vi "ASCII_To_Hex.vi"(11 "ASCII String":string) -> (0 "hex 4":u8, 1 "hex 3":u8, 2 "hex 2":u8, 3 "hex1":u8, 5 "hex数组":u16[](array[numeric]) format="%x")   [LabVIEW 2018]
panel:
  out "hex5":u8
  out "hex6":u8
  out "hex 7":u8
  out "hex 8":u8
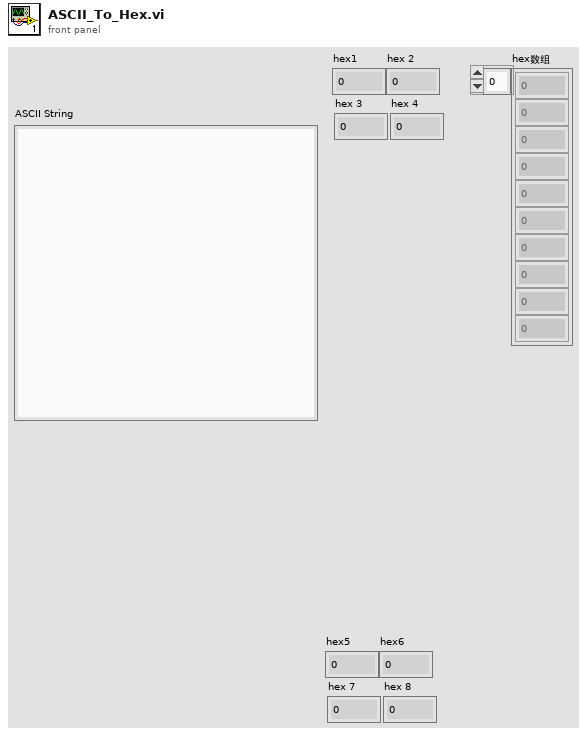
[diagram p1: front panel]
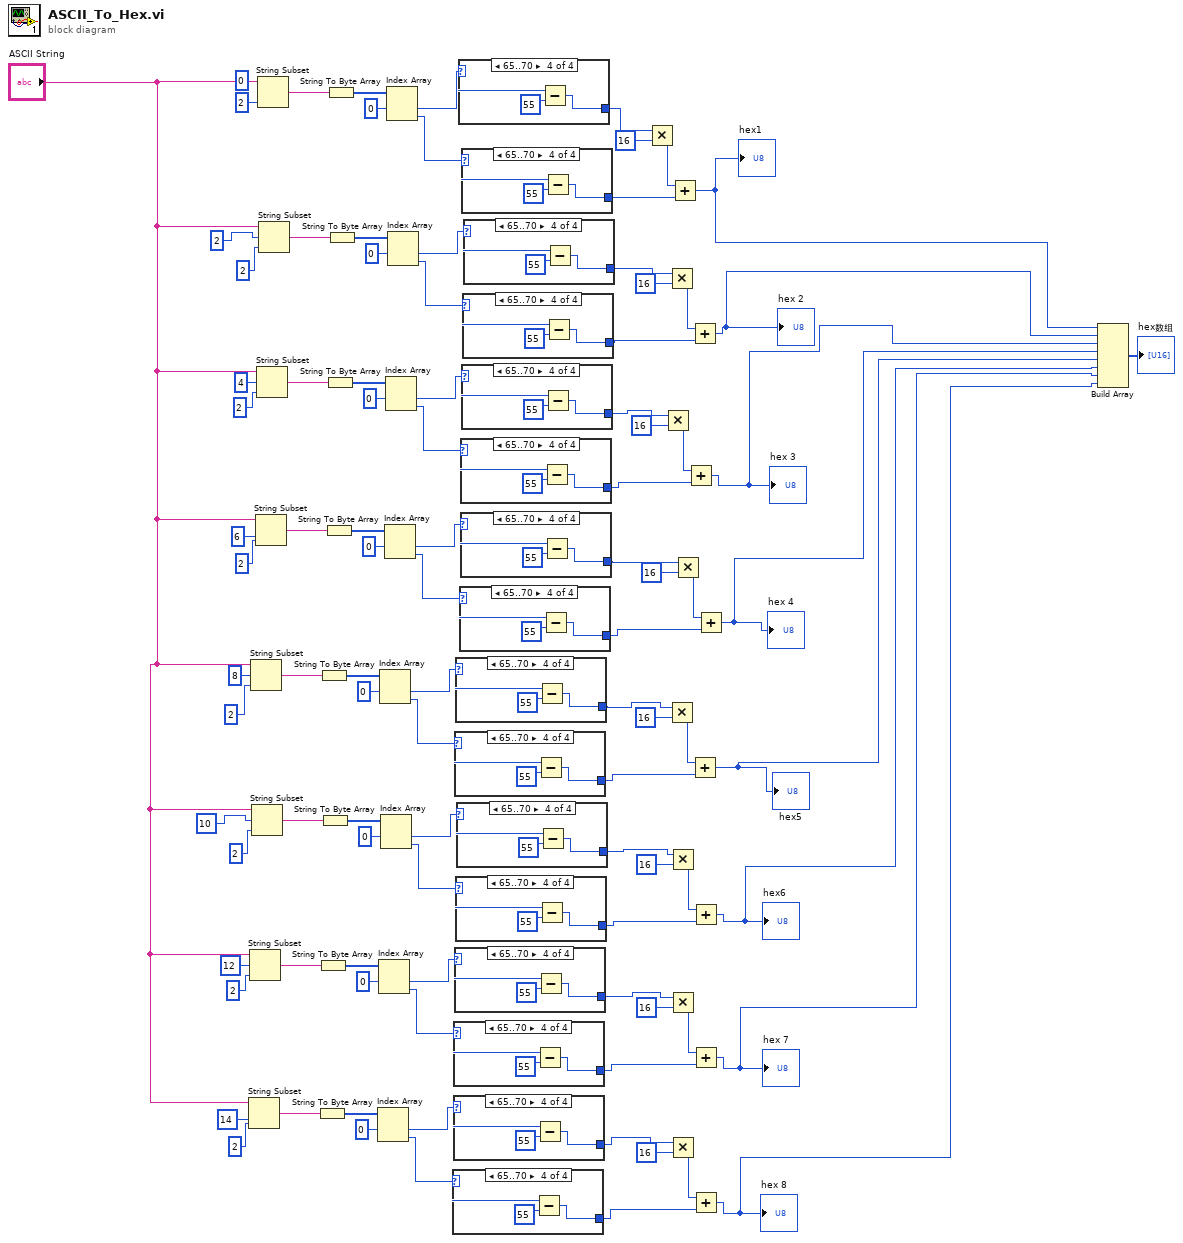
[diagram p0: block diagram]
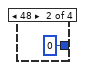
[diagram p3: hidden frame]
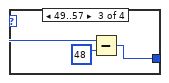
[diagram p4: hidden frame]
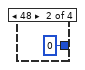
[diagram p6: hidden frame]
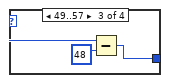
[diagram p7: hidden frame]
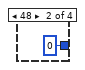
[diagram p9: hidden frame]
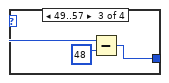
[diagram p10: hidden frame]
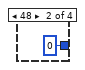
[diagram p12: hidden frame]
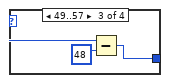
[diagram p13: hidden frame]
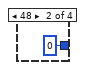
[diagram p15: hidden frame]
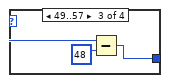
[diagram p16: hidden frame]
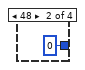
[diagram p18: hidden frame]
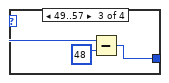
[diagram p19: hidden frame]
diagram:
  n1 = String Subset(string="ASCII String", offset (0)=14 ("偏移量(0)"), length (rest)=2 ("长度（剩余）")) -> (substring=w67:string)
  n2 = String Subset(string="ASCII String", offset (0)=12 ("偏移量(0)"), length (rest)=2 ("长度（剩余）")) -> (substring=w58:string)
  n3 = String Subset(string="ASCII String", offset (0)=8 ("偏移量(0)"), length (rest)=2 ("长度（剩余）")) -> (substring=w46:string)
  n4 = String Subset(string="ASCII String", offset (0)=10 ("偏移量(0)"), length (rest)=2 ("长度（剩余）")) -> (substring=w55:string)
  n5 = String Subset(string="ASCII String", offset (0)=6 ("偏移量(0)"), length (rest)=2 ("长度（剩余）")) -> (substring=w76:string)
  n6 = String Subset(string="ASCII String", offset (0)=4 ("偏移量(0)"), length (rest)=2 ("长度（剩余）")) -> (substring=w85:string)
  n7 = String Subset(string="ASCII String", offset (0)=0 ("偏移量(0)"), length (rest)=2 ("长度（剩余）")) -> (substring=w97:string)
  n8 = String Subset(string="ASCII String", offset (0)=2 ("偏移量(0)"), length (rest)=2 ("长度（剩余）")) -> (substring=w88:string)
  n9 = String To Byte Array(string=w67) -> (unsigned byte array=w66:u8[])
  n10 = String To Byte Array(string=w58) -> (unsigned byte array=w59:u8[])
  n11 = String To Byte Array(string=w46) -> (unsigned byte array=w47:u8[])
  n12 = String To Byte Array(string=w55) -> (unsigned byte array=w54:u8[])
  n13 = String To Byte Array(string=w76) -> (unsigned byte array=w77:u8[])
  n14 = String To Byte Array(string=w85) -> (unsigned byte array=w84:u8[])
  n15 = String To Byte Array(string=w97) -> (unsigned byte array=w96:u8[])
  n16 = String To Byte Array(string=w88) -> (unsigned byte array=w89:u8[])
  n17 = Index Array(array=w66, index #1=0 ("索引")) -> (element #1=w64:u8, element #2=w63:u8)  [unwired: 1 in]
  n18 = Index Array(array=w59, index #1=0 ("索引")) -> (element #1=w61:u8, element #2=w62:u8)  [unwired: 1 in]
  n19 = Index Array(array=w47, index #1=0 ("索引")) -> (element #1=w49:u8, element #2=w50:u8)  [unwired: 1 in]
  n20 = Index Array(array=w54, index #1=0 ("索引")) -> (element #1=w52:u8, element #2=w51:u8)  [unwired: 1 in]
  n21 = Index Array(array=w77, index #1=0 ("索引")) -> (element #1=w79:u8, element #2=w80:u8)  [unwired: 1 in]
  n22 = Index Array(array=w84, index #1=0 ("索引")) -> (element #1=w82:u8, element #2=w81:u8)  [unwired: 1 in]
  n23 = Index Array(array=w96, index #1=0 ("索引")) -> (element #1=w94:u8, element #2=w93:u8)  [unwired: 1 in]
  n24 = Index Array(array=w89, index #1=0 ("索引")) -> (element #1=w91:u8, element #2=w92:u8)  [unwired: 1 in]
  n25 = case shown="65..70" w63 {
    selector: w63 -> [w99 _ w103 w106]
    tunnel: [w99 u8 0 w101 w104] -> w9
    frame 0, Default {
    }
    frame 48 {
    }
    frame 49..57 {
      n26 = Subtract(x=w103, y=u8 48) -> (x-y=w101:u8)
    }
    frame 65..70 {
      n27 = Subtract(x=w106, y=u8 55) -> (x-y=w104:u8)
    }
  }
  n28 = case shown="65..70" w62 {
    selector: w62 -> [w107 _ w111 w114]
    tunnel: [w107 u8 0 w109 w112] -> w11
    frame 0, Default {
    }
    frame 48 {
    }
    frame 49..57 {
      n29 = Subtract(x=w111, y=u8 48) -> (x-y=w109:u8)
    }
    frame 65..70 {
      n30 = Subtract(x=w114, y=u8 55) -> (x-y=w112:u8)
    }
  }
  n31 = case shown="65..70" w64 {
    selector: w64 -> [w115 _ w119 w122]
    tunnel: [w115 u8 0 w117 w120] -> w10
    frame 0, Default {
    }
    frame 48 {
    }
    frame 49..57 {
      n32 = Subtract(x=w119, y=u8 48) -> (x-y=w117:u8)
    }
    frame 65..70 {
      n33 = Subtract(x=w122, y=u8 55) -> (x-y=w120:u8)
    }
  }
  n34 = case shown="65..70" w50 {
    selector: w50 -> [w123 _ w127 w130]
    tunnel: [w123 u8 0 w125 w128] -> w15
    frame 0, Default {
    }
    frame 48 {
    }
    frame 49..57 {
      n35 = Subtract(x=w127, y=u8 48) -> (x-y=w125:u8)
    }
    frame 65..70 {
      n36 = Subtract(x=w130, y=u8 55) -> (x-y=w128:u8)
    }
  }
  n37 = case shown="65..70" w61 {
    selector: w61 -> [w131 _ w135 w138]
    tunnel: [w131 u8 0 w133 w136] -> w12
    frame 0, Default {
    }
    frame 48 {
    }
    frame 49..57 {
      n38 = Subtract(x=w135, y=u8 48) -> (x-y=w133:u8)
    }
    frame 65..70 {
      n39 = Subtract(x=w138, y=u8 55) -> (x-y=w136:u8)
    }
  }
  n40 = case shown="65..70" w49 {
    selector: w49 -> [w139 _ w143 w146]
    tunnel: [w139 u8 0 w141 w144] -> w16
    frame 0, Default {
    }
    frame 48 {
    }
    frame 49..57 {
      n41 = Subtract(x=w143, y=u8 48) -> (x-y=w141:u8)
    }
    frame 65..70 {
      n42 = Subtract(x=w146, y=u8 55) -> (x-y=w144:u8)
    }
  }
  n43 = case shown="65..70" w51 {
    selector: w51 -> [w147 _ w151 w154]
    tunnel: [w147 u8 0 w149 w152] -> w13
    frame 0, Default {
    }
    frame 48 {
    }
    frame 49..57 {
      n44 = Subtract(x=w151, y=u8 48) -> (x-y=w149:u8)
    }
    frame 65..70 {
      n45 = Subtract(x=w154, y=u8 55) -> (x-y=w152:u8)
    }
  }
  n46 = case shown="65..70" w52 {
    selector: w52 -> [w155 _ w159 w162]
    tunnel: [w155 u8 0 w157 w160] -> w14
    frame 0, Default {
    }
    frame 48 {
    }
    frame 49..57 {
      n47 = Subtract(x=w159, y=u8 48) -> (x-y=w157:u8)
    }
    frame 65..70 {
      n48 = Subtract(x=w162, y=u8 55) -> (x-y=w160:u8)
    }
  }
  n49 = case shown="65..70" w94 {
    selector: w94 -> [w163 _ w167 w170]
    tunnel: [w163 u8 0 w165 w168] -> w39
    frame 0, Default {
    }
    frame 48 {
    }
    frame 49..57 {
      n50 = Subtract(x=w167, y=u8 48) -> (x-y=w165:u8)
    }
    frame 65..70 {
      n51 = Subtract(x=w170, y=u8 55) -> (x-y=w168:u8)
    }
  }
  n52 = case shown="65..70" w80 {
    selector: w80 -> [w171 _ w175 w178]
    tunnel: [w171 u8 0 w173 w176] -> w17
    frame 0, Default {
    }
    frame 48 {
    }
    frame 49..57 {
      n53 = Subtract(x=w175, y=u8 48) -> (x-y=w173:u8)
    }
    frame 65..70 {
      n54 = Subtract(x=w178, y=u8 55) -> (x-y=w176:u8)
    }
  }
  n55 = case shown="65..70" w81 {
    selector: w81 -> [w179 _ w183 w186]
    tunnel: [w179 u8 0 w181 w184] -> w19
    frame 0, Default {
    }
    frame 48 {
    }
    frame 49..57 {
      n56 = Subtract(x=w183, y=u8 48) -> (x-y=w181:u8)
    }
    frame 65..70 {
      n57 = Subtract(x=w186, y=u8 55) -> (x-y=w184:u8)
    }
  }
  n58 = case shown="65..70" w79 {
    selector: w79 -> [w187 _ w191 w194]
    tunnel: [w187 u8 0 w189 w192] -> w18
    frame 0, Default {
    }
    frame 48 {
    }
    frame 49..57 {
      n59 = Subtract(x=w191, y=u8 48) -> (x-y=w189:u8)
    }
    frame 65..70 {
      n60 = Subtract(x=w194, y=u8 55) -> (x-y=w192:u8)
    }
  }
  n61 = case shown="65..70" w93 {
    selector: w93 -> [w195 _ w199 w202]
    tunnel: [w195 u8 0 w197 w200] -> w41
    frame 0, Default {
    }
    frame 48 {
    }
    frame 49..57 {
      n62 = Subtract(x=w199, y=u8 48) -> (x-y=w197:u8)
    }
    frame 65..70 {
      n63 = Subtract(x=w202, y=u8 55) -> (x-y=w200:u8)
    }
  }
  n64 = case shown="65..70" w82 {
    selector: w82 -> [w203 _ w207 w210]
    tunnel: [w203 u8 0 w205 w208] -> w20
    frame 0, Default {
    }
    frame 48 {
    }
    frame 49..57 {
      n65 = Subtract(x=w207, y=u8 48) -> (x-y=w205:u8)
    }
    frame 65..70 {
      n66 = Subtract(x=w210, y=u8 55) -> (x-y=w208:u8)
    }
  }
  n67 = case shown="65..70" w92 {
    selector: w92 -> [w211 _ w215 w218]
    tunnel: [w211 u8 0 w213 w216] -> w21
    frame 0, Default {
    }
    frame 48 {
    }
    frame 49..57 {
      n68 = Subtract(x=w215, y=u8 48) -> (x-y=w213:u8)
    }
    frame 65..70 {
      n69 = Subtract(x=w218, y=u8 55) -> (x-y=w216:u8)
    }
  }
  n70 = case shown="65..70" w91 {
    selector: w91 -> [w219 _ w223 w226]
    tunnel: [w219 u8 0 w221 w224] -> w22
    frame 0, Default {
    }
    frame 48 {
    }
    frame 49..57 {
      n71 = Subtract(x=w223, y=u8 48) -> (x-y=w221:u8)
    }
    frame 65..70 {
      n72 = Subtract(x=w226, y=u8 55) -> (x-y=w224:u8)
    }
  }
  n73 = Multiply(x=w39, y=u8 16) -> (x*y=w37:u8)
  n74 = Multiply(x=w20, y=u8 16) -> (x*y=w33:u8)
  n75 = Multiply(x=w22, y=u8 16) -> (x*y=w36:u8)
  n76 = Multiply(x=w16, y=u8 16) -> (x*y=w29:u8)
  n77 = Multiply(x=w14, y=u8 16) -> (x*y=w28:u8)
  n78 = Multiply(x=w12, y=u8 16) -> (x*y=w25:u8)
  n79 = Multiply(x=w10, y=u8 16) -> (x*y=w24:u8)
  n80 = Add(x=w37, y=w41) -> (x+y=w40:u8)
  "hex1" <- w40
  n81 = Multiply(x=w18, y=u8 16) -> (x*y=w32:u8)
  n82 = Add(x=w33, y=w19) -> (x+y=w7:u8)
  "hex 3" <- w7
  n83 = Add(x=w36, y=w21) -> (x+y=w8:u8)
  "hex 2" <- w8
  n84 = Add(x=w29, y=w15) -> (x+y=w5:u8)
  "hex5" <- w5
  n85 = Add(x=w28, y=w13) -> (x+y=w4:u8)
  "hex6" <- w4
  n86 = Add(x=w25, y=w11) -> (x+y=w3:u8)
  "hex 7" <- w3
  n87 = Add(x=w24, y=w9) -> (x+y=w2:u8)
  "hex 8" <- w2
  n88 = Add(x=w32, y=w17) -> (x+y=w6:u8)
  "hex 4" <- w6
  n89 = Build Array(w40, w8, w7, w6, w5, w4, w3, w2) -> (→"hex数组":u8[])
